vi "Year2019 Q2.vi"() -> ()   [LabVIEW 2018]
panel:
  out "Counter":dbl
  in  "Reset":bool
  in  "Count down":bool
  in  "Count up":bool
  in  "Run":bool
  # "Press this 'Run\" first\nbefore pressing the\n\"Arrow\" on top panel"
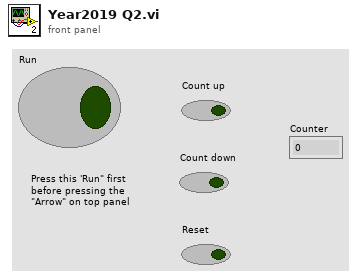
[diagram p1: front panel]
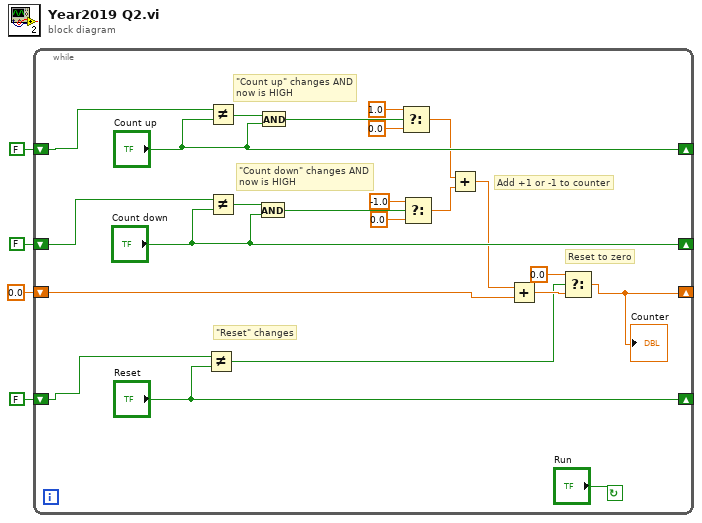
[diagram p0: block diagram]
diagram:
  n1 = while {
    shift-right: ["Count up"] -> _
    shift-left: FALSE ("Count up") -> [w26]
    shift-right: ["Count down"] -> _
    shift-left: FALSE ("Count down") -> [w23]
    shift-right: ["Reset"] -> _
    shift-left: FALSE ("Reset") -> [w7]
    shift-right: [w5] -> _
    shift-left: 0.0 ("t") -> [w11]
    stop <- "Run" continue-if-true
    # "Reset to zero"
    # "Add +1 or -1 to counter"
    # "\"Reset\" changes"
    # "\"Count down\" changes AND\nnow is HIGH"
    # "\"Count up\" changes AND\nnow is HIGH"
    n2 = Not Equal?(x=w7, y="Reset") -> (x != y?=w6:bool)
    n3 = Not Equal?(x=w26, y="Count up") -> (x != y?=w25:bool)
    n4 = Not Equal?(x=w23, y="Count down") -> (x != y?=w22:bool)
    n5 = And(x=w22, y="Count down") -> (x .and. y?=w18:bool)
    n6 = And(x=w25, y="Count up") -> (x .and. y?=w20:bool)
    n7 = Select(t=1.0, s=w20, f=0.0) -> (s? t:f=w13:dbl)
    n8 = Select(t=-1.0, s=w18, f=0.0) -> (s? t:f=w14:dbl)
    n9 = Add(x=w13, y=w14) -> (x+y=w12:dbl)
    n10 = Add(x=w12, y=w11) -> (x+y=w10:dbl)
    n11 = Select(t=0.0, s=w6, f=w10) -> (s? t:f=w5:dbl)
    "Counter" <- w5
  }
